vi "UDP - Sender.vi"(7 "destination address":string="255.255.255.255", 8 "error in (no error)":errorcluster, 10 "remote port":u16=61557, 11 "port":u16=61556) -> (0 "error out":errorcluster, 2 "current value":dbl, 3 "Array Out":dbl[](array[numeric]))   [LabVIEW 2019]
doc: "The UDP protocol differs from TCP in that there is no error-checking with the packets of information that are sent, and thus no guarantee whatsoever that an intended recipient will actually receive a given piece of data.\n\nUDP does offer the ability to \"broadcast\" data across a network--simply specify an IP Address of all ones (255.255.255.255) to attempt to broadcast information network-wide. Keep in mind that routers and other network hardware will generally refuse to forward the broadcast beyond certain points, so the extent of the broadcast will in practice be limited."
panel:
  # "Overview: Sends UDP data to the destination addresses. Set destination address to the server address or to 255.255.255.255 to send to the entire network.\n\nInstructions:\n1. Run the VI and click Start Test\n2. Open Simple UDP - Receiver.vi and follow the instructions on its front panel.\n3. Click Stop to stop the VI."
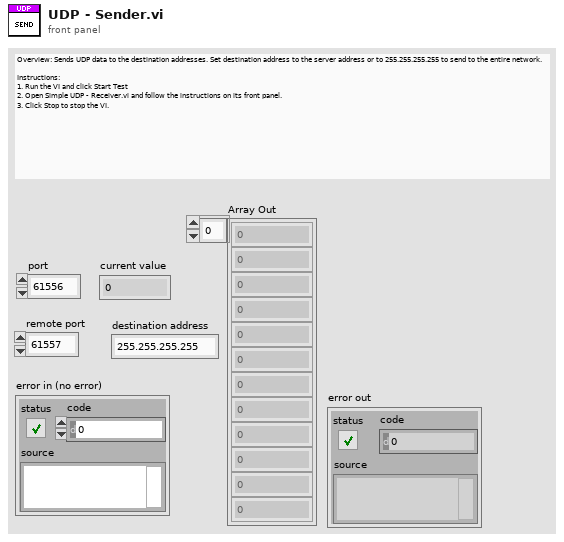
[diagram p1: front panel]
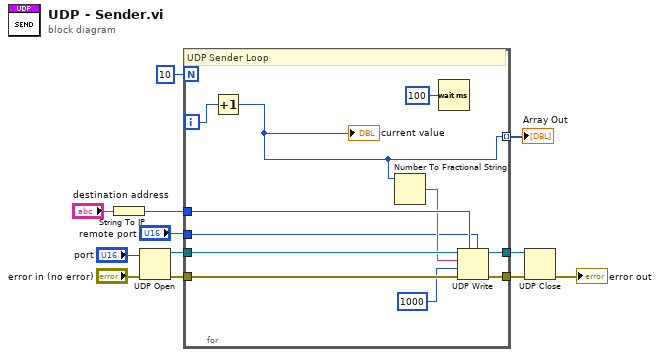
[diagram p0: block diagram]
diagram:
  n1 = String To IP(1:"destination address") -> (0:w7:u32)
  n2 = UDP Open(8:"error in (no error)", 11:"port") -> (port=w6:refnum<k16>, 0:w5:errorcluster)  [unwired: 3 in, 1 out]
  n3 = for {
    N: 10 -> [_]
    tunnel: [w17] -> w9
    tunnel: w6 -> [w23]
    tunnel: w5 -> [w22]
    tunnel: [w21] -> w10
    tunnel: w7 -> [w20]
    tunnel: "remote port" -> [w15]
    tunnel: [w14] -> w2 mode=indexing
    i -> [w13]
    # "UDP Sender Loop"
    n4 = Increment(x=w13) -> (x+1=w14:i32)
    "current value" <- w14
    n5 = Number To Fractional String(number=w14) -> (F-format string=w18:string)  [unwired: 3 in]
    n6 = Wait (ms)(milliseconds to wait=u32 100) -> ()  [unwired: 1 out]
    n7 = UDP Write(address=w20, port or service name=w15, connection ID=w23, data in=w18, 8:w22, 9:1000 ("timeout ms (25000)")) -> (error out=w17:errorcluster, 3:w21:refnum<k16>)
  }
  "Array Out" <- w2
  n8 = UDP Close(connection ID=w10, 8:w9) -> (error out=→"error out":errorcluster)  [unwired: 1 out]
